vi "resetHP.vi"(0 "ILCCommunications in":refnum<class "ILCCommunications.lvclass">, 5 "HPIndex":i32, 7 "WaitForTrigger":bool, 9 "TriggerIRQ":bool, 11 "error in (no error)":errorcluster) -> (4 "ILCCommunications out":refnum<class "ILCCommunications.lvclass">, 15 "error out":errorcluster)   [LabVIEW 2016, in "ILCCommunications.lvclass"]
uses:
  ILCCommunications.lvclass
  ILCCommunications.lvclass/ILCCommunications.ctl
  Common_RT_HPILC/HPILC/HPILC.lvclass
  D:/Code/ts_M1M3Support/Common_RT_ILC/ILC/ILC.lvclass
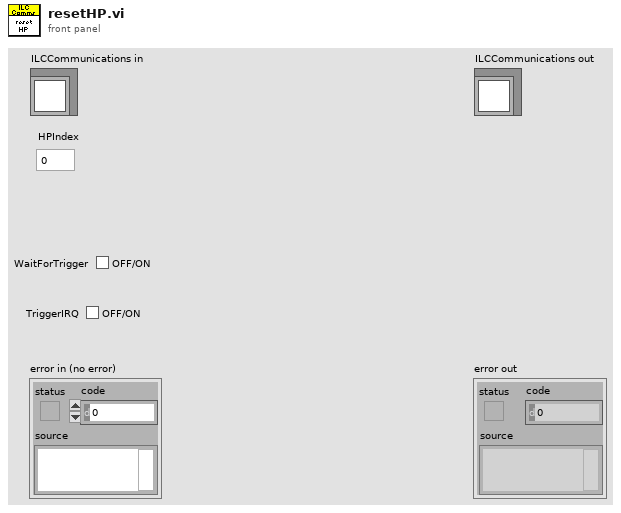
[diagram p1: front panel]
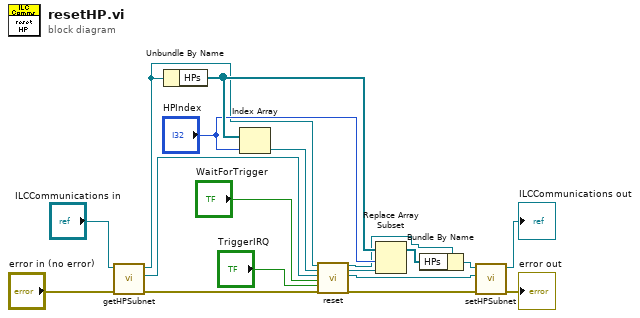
[diagram p0: block diagram]
diagram:
  n1 = call "getHPSubnet.vi"("error in (no error)"="error in (no error)", "ILCCommunications in"="ILCCommunications in") -> ("error out"=w8:errorcluster, "Modbus"=w4:refnum<class "IModbus.lvclass">, "ILCCommunications out"=w10:refnum<class "ILCCommunications.lvclass">)  [unwired: 7 in]
  n2 = Unbundle By Name(w10) -> ("HPs"=w18:refnum<class "HPILC.lvclass">[])
  n3 = Index Array(array=w18, index="HPIndex") -> (element=w1:refnum<class "HPILC.lvclass">)
  n4 = call "reset.vi"("ILCCommunications in"=w10, "ILC in"=w1, "Modbus in"=w4, "WaitForTrigger"="WaitForTrigger", "TriggerIRQ"="TriggerIRQ", "error in (no error)"=w8) -> ("ILCCommunications out"=w9:refnum<class "ILCCommunications.lvclass">, "ILC out"=w2:refnum<class "HPILC.lvclass">, "Modbus out"=w3:refnum<class "IModbus.lvclass">, "error out"=w7:errorcluster)  [unwired: 10 in]
  n5 = Replace Array Subset(array=w18, new element=w2, index="HPIndex") -> (w17:refnum<class "HPILC.lvclass">[])
  n6 = Bundle By Name(cluster=w9, "HPs"=w17) -> (w12:refnum<class "ILCCommunications.lvclass">)
  n7 = call "setHPSubnet.vi"("error in (no error)"=w7, "Modbus"=w3, "ILCCommunications in"=w12) -> ("error out"=→"error out":errorcluster, "ILCCommunications out"=→"ILCCommunications out":refnum<class "ILCCommunications.lvclass">)  [unwired: 7 in]
